vi "Get Decimation.vi"(8 "error in":errorcluster, 11 "custom device ref":T1 format="%.0x") -> (0 "error out":errorcluster, 2 "Decimation":i32, 3 "custom device ref out":T1 format="%.0x")   [LabVIEW 2020, in "AIM ARINC 429 Scripting.lvlib"]
doc: "Reads the <b>description</b> field of the input <b>AIM ARINC 429 custom device</b>."
uses:
  <vilib>/NI VeriStand/Custom Device API/Custom Device Item Ref.ctl
  AIM ARINC 429 Scripting.lvlib
  <vilib>/NI VeriStand/Custom Device API/Custom Device API.lvlib
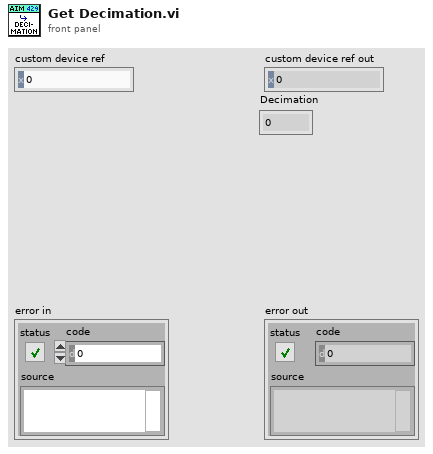
[diagram p1: front panel]
types:
  T1 = typedef "Custom Device API.lvlib/Custom Device Item Ref.ctl" = u64
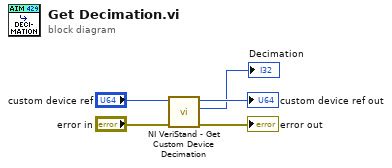
[diagram p0: block diagram]
diagram:
  n1 = call <vilib>:"NI VeriStand - Get Custom Device Decimation.vi"("error in (no error)"="error in", "Device Ref in"="custom device ref") -> ("error out"=→"error out":errorcluster, "Decimation"=→"Decimation":i32, "Device Ref out"=→"custom device ref out":T1)  [unwired: 7 in]
